vi "GEM_BANK_ARRAY_Get_N_Banks.vi"(8 "error in (no error)":errorcluster, 11 "GEM_BANK_ARRAY in":refnum<class "GEM_BANK_ARRAY.lvclass">) -> (0 "error out":errorcluster, 2 "Array Size":i32, 3 "GEM_BANK_ARRAY out":refnum<class "GEM_BANK_ARRAY.lvclass">)   [LabVIEW 2018, in "feGEM DataPacker.lvlib" / "GEM_BANK_ARRAY.lvclass"]
uses:
  GEM_BANK_ARRAY.lvclass
  GEM_BANK_ARRAY.lvclass/GEM_BANK_ARRAY.ctl
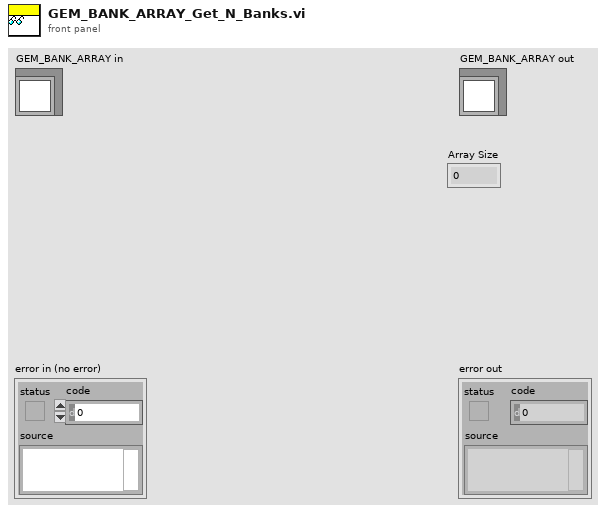
[diagram p1: front panel]
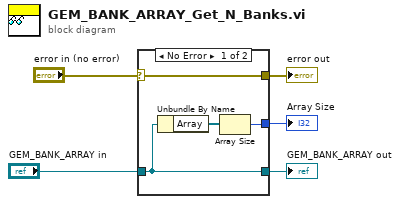
[diagram p0: block diagram]
diagram:
  n1 = case shown="No Error" "error in (no error)" {
    selector: "error in (no error)" -> [w9 w10]
    tunnel: [w9 w10] -> w4
    tunnel: [w8 w11] -> w2
    tunnel: "GEM_BANK_ARRAY in" -> [w8 w11]
    tunnel: [w7 _] -> w1
    frame No Error {
      n2 = Unbundle By Name(w8) -> ("Array"=w6:refnum<class "GEM_BANK.lvclass">[])
      n3 = Array Size(array=w6) -> (size(s)=w7:i32)
    }
    frame Error {
    }
  }
  "error out" <- w4
  "GEM_BANK_ARRAY out" <- w2
  "Array Size" <- w1
